vi "Launcher.vi"() -> ()   [LabVIEW 2015]
uses:
  Inspection Statemachine/Inspection Statemachine.lvclass
  <vilib>/ActorFramework/Actor/Actor.lvclass
panel:
  out "error out":errorcluster
  in  "error in (no error)":errorcluster
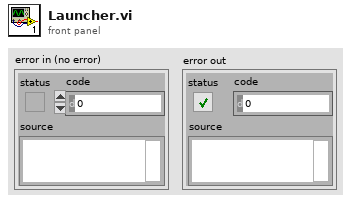
[diagram p1: front panel]
types:
  T1 = cluster{"Operation Mode":string, "Product Name":string, "Company Name":string, "Batch Number":string}
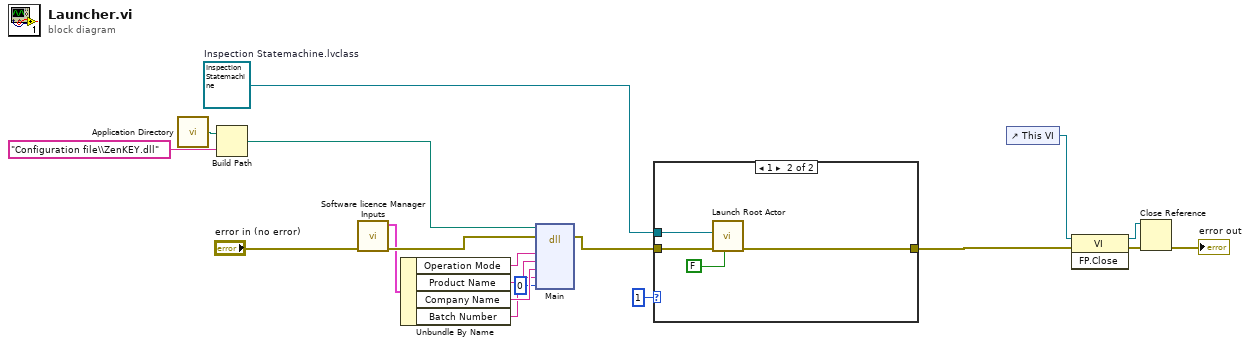
[diagram p0: block diagram]
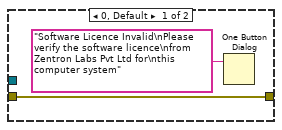
[diagram p2: hidden frame]
diagram:
  w17 = refnum<class "Inspection Statemachine.lvclass"> refnum  # Inspection Statemachine.lvclass
  n1 = call <vilib>:"Application Directory.vi"() -> ("Application Directory"=w12:path)
  n2 = Build Path(base path=w12, name or relative path="Configuration file\\ZenKEY.dll") -> (appended path=w10:path)
  n3 = call "Software licence Manager Inputs.vi"("error in (no error)"="error in (no error)") -> ("error out"=w8:errorcluster, "Software Licence Manager Inputs Out"=w7:T1)  [unwired: 9 in]
  n4 = Unbundle By Name(w7) -> ("Operation Mode"=w6:string, "Product Name"=w5:string, "Company Name"=w4:string, "Batch Number"=w3:string)
  n5 = dll-call lib="C:/Users/raakeshs/Desktop/ZenGage V1.2/Configuration file/ZenKEY.dll" fn="Main"(path in=w10, error in=w8, "operationMode"=w6, "projectName"=w5, "customerName"=w4, "batchNumber"=w3, "result"=u8 0) -> (error out=w13:errorcluster)  [unwired: 7 in, 1 out]
  n6 = case shown="1" u8 1 ("result") {
    tunnel: [w20 w25] -> w18
    tunnel: w17 -> [_ w24]
    tunnel: w13 -> [w20 w22]
    frame 0, Default {
      n7 = One Button Dialog(message="Software Licence Invalid\nPlease verify the software licence\nfrom Zentron Labs Pvt Ltd for\nthis computer system") -> ()  [unwired: 1 in, 1 out]
    }
    frame 1 {
      n8 = call <vilib>:"Launch Root Actor.vi"("Open Actor Core front panel? (F)"=FALSE, "error in (no error)"=w22, "Actor"=w24) -> ("error out"=w25:errorcluster)  [unwired: 7 in, 1 out]
    }
  }
  n9 = control-ref of="This VI"() -> (w19:refnum<vi>)
  n10 = invoke class="VI" method="FP.Close"(reference=w19, error in=w18) -> (reference out=w15:refnum<vi>, error out=w16:errorcluster)  [unwired: 1 in, 1 out]
  n11 = Close Reference(reference=w15, error in (no error)=w16) -> (error out=→"error out":errorcluster)
